vi "LM IRF(X)PSED and gradient v4.vi"(3 "output control":T1, 4 "data":variant, 5 "X":dbl[](array[numeric]), 6 "a":dbl[](array[numeric])) -> (0 "error out":errorcluster, 1 "f'(X,a)":dbl[][](array[numeric]), 2 "f(X,a)":dbl[](array[numeric]))   [LabVIEW 2019]
doc: "This template is the starting point for creating a model function to be passed to the Nonlinear Curve Fit.vi."
uses:
  <vilib>/gmath/NumericalOptimization/LM_output select.ctl
  <vilib>/gmath/NI_Gmath.lvlib
panel:
  # "Parameters:\n\nb"
  # "Data:\n\ntau, IRF order, T, {Ck, Sk, phi_k, epsilon_k}"
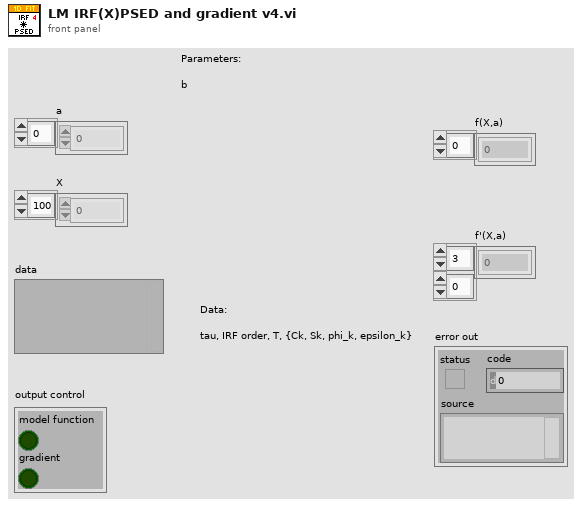
[diagram p1: front panel]
types:
  T1 = typedef "NI_Gmath.lvlib/LM_output select.ctl" = cluster{"model function":bool, "gradient":bool}
  T2 = typedef "IRF(X)PSED Fixed Parameters v3.ctl" = cluster{"order":i32, "T":dbl, "Time Constant Array":dbl[], "{S_k, C_k, phi_k, e_k} arrays":cluster{"S_k Array":dbl[], "C_k Array":dbl[], "phi_k Array":dbl[], "e_k Array":dbl[]}, "IRF Extraction Options":T3}
  T3 = typedef "IRF(X)PSED Extraction Options.ctl" = cluster{"Time Constant for IRF Extraction":dbl[unit], "IRF Order":i32, "Fourier Series Smoothing":T4, "Noise Threshold":dbl, "Smoothing Width":dbl, "Fourier Series Truncation":T5, "Truncation Order":i32, "Save Power Spectrum":bool}
  T4 = typedef "Fourier Series Smoothing Option.ctl" = enum16{"None", "Lanczos Factors", "Fejer Summation"}
  T5 = typedef "Fourier Series Truncation.ctl" = enum16{"Automatic", "Fixed"}
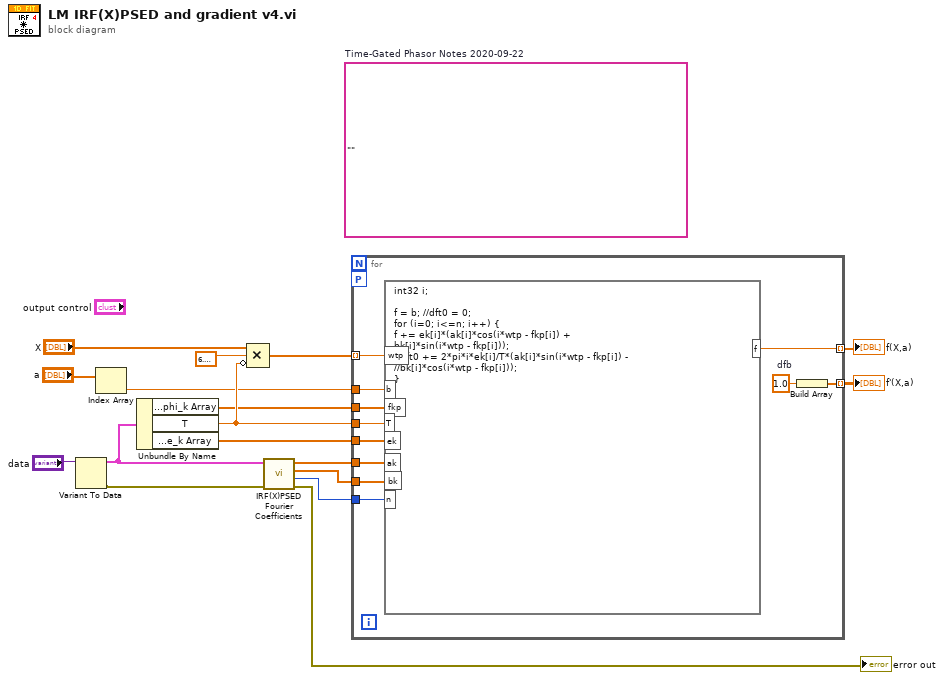
[diagram p0: block diagram]
diagram:
  (unwired) ""  # Time-Gated Phasor Notes 2020-09-22
  n1 = Variant To Data(Variant="data") -> (data=w6:T2, error out=w3:errorcluster)  [unwired: 2 in]
  n2 = Index Array(array="a") -> (element=w9:dbl)  [unwired: 1 in]
  n3 = Unbundle By Name(w6) -> ("{S_k, C_k, phi_k, e_k} arrays.phi_k Array"=w8:dbl[], "T"=w10:dbl, "{S_k, C_k, phi_k, e_k} arrays.e_k Array"=w7:dbl[])
  n4 = Compound Arithmetic op=MULTIPLY("X", 6.283185307179586, invert w10) -> (w11:dbl[])
  n5 = call "IRF(X)PSED Fourier Coefficients.vi"("Error In"=w3, "IRF*PSED fixed Parameters"=w6) -> ("Error Out"=→"error out":errorcluster, "Optimal Order"=w1:i32, "[b_k]"=w4:dbl[], "[a_k]"=w5:dbl[])  [unwired: 4 in, 2 out]
  n6 = for {
    tunnel: w11 -> [w28] mode=indexing
    tunnel: [w27] -> w17 mode=indexing
    tunnel: [w26] -> w14 mode=indexing
    tunnel: w9 -> [w25]
    tunnel: w1 -> [w24]
    tunnel: w5 -> [w21]
    tunnel: w4 -> [w20]
    tunnel: w8 -> [w22]
    tunnel: w10 -> [w19]
    tunnel: w7 -> [w18]
    workers-P: _ -> [_]
    w23 = 1.0  # dfb
    n7 = formula code="int32 i;\n\nf = b; //dft0 = 0;\nfor (i=0; i<=n; i++) {\nf += ek[i]*(ak[i]*cos(i*wtp - fkp[i]) +\nbk[i]*sin(i*wtp - fkp[i]));\n//dft0 += 2*pi*i*ek[i]/T*(ak[i]*sin(i*wtp - fkp[i]) -\n//bk[i]*cos(i*wtp - fkp[i]));\n}"("wtp"=w28, "b"=w25, "n"=w24, "fkp"=w22, "ak"=w21, "bk"=w20, "T"=w19, "ek"=w18) -> ("f"=w27:dbl)
    n8 = Build Array(w23) -> (w26:dbl[])
  }
  "f(X,a)" <- w17
  "f'(X,a)" <- w14
